vi "Utility Format Flow Rate.vi"(8 "error in (no error)":errorcluster, 11 "Flow Rate":dbl) -> (0 "error out":errorcluster, 3 "Formatted Flow Rate":string)   [LabVIEW 2020, in "driver_chromtech_nextgen_pump.lvlib"]
uses:
  driver_chromtech_nextgen_pump.lvlib
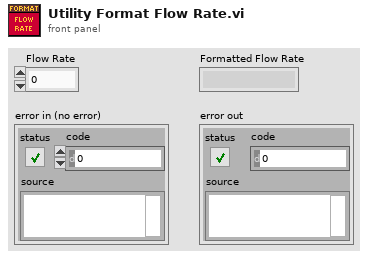
[diagram p1: front panel]
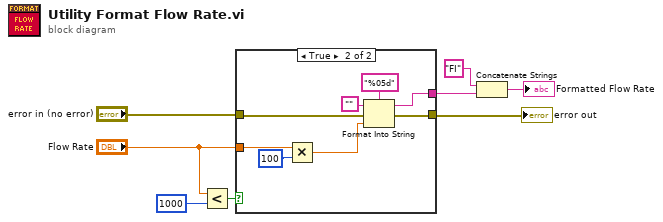
[diagram p0: block diagram]
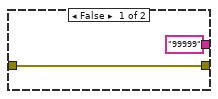
[diagram p2: hidden frame]
diagram:
  n1 = Less?(x="Flow Rate", y=1000) -> (x < y?=w6:bool)
  n2 = case shown="True" w6 {
    tunnel: "error in (no error)" -> [w10 w17]
    tunnel: "Flow Rate" -> [_ w13]
    tunnel: [w10 w16] -> w5
    tunnel: ["99999" w15] -> w1
    frame False {
    }
    frame True {
      n3 = Multiply(x=w13, y=100) -> (x*y=w12:dbl)
      n4 = Format Into String(format string="%05d", initial string="", error in=w17, w12) -> (resulting string=w15:string, error out=w16:errorcluster)
    }
  }
  "error out" <- w5
  n5 = Concatenate Strings("FI", w1) -> (→"Formatted Flow Rate":string)
